vi "Begin routeguide_RouteGuide_RouteChat.vi"(8 "error in":errorcluster, 9 "contextId":T1, 11 "gRPC ID":T1) -> (0 "error out":errorcluster, 2 "Call Id Out":T1, 3 "gRPC ID out":T1)   [LabVIEW 2019, in "route_guide_client.lvlib"]
uses:
  route_guide_client.lvlib
  <vilib>/gRPC/LabVIEW gRPC Library/Shared/grpcId.ctl
  <vilib>/gRPC/LabVIEW gRPC Library/grpc-lvsupport-release.lvlib
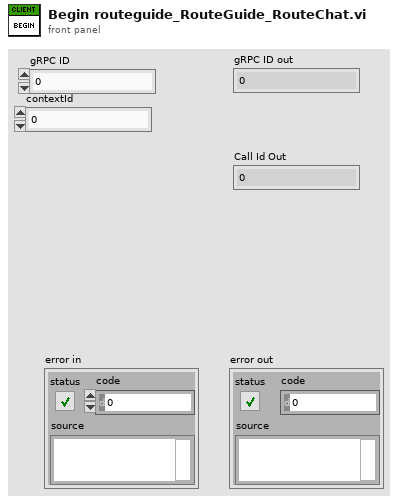
[diagram p1: front panel]
types:
  T1 = typedef "grpc-lvsupport-release.lvlib/grpcId.ctl" = u64
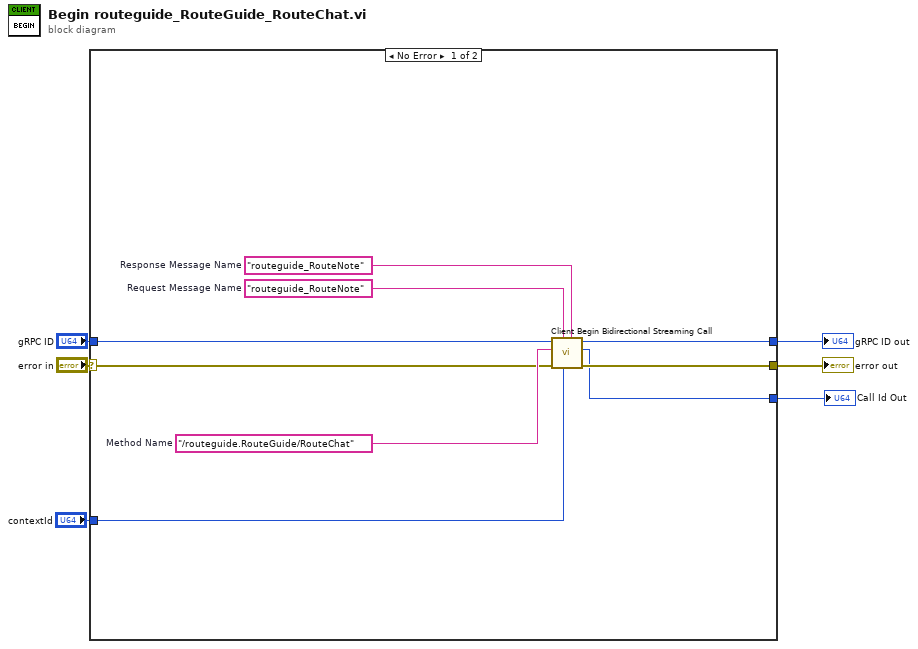
[diagram p0: block diagram]
diagram:
  n1 = case shown="No Error" "error in" {
    selector: "error in" -> [w12 w16]
    tunnel: [w11 w16] -> w5
    tunnel: "gRPC ID" -> [w10 w17]
    tunnel: [w9 w17] -> w3
    tunnel: [w8 _] -> w2
    tunnel: "contextId" -> [w7 _]
    frame No Error {
      w13 = "routeguide_RouteNote"  # Response Message Name
      w14 = "routeguide_RouteNote"  # Request Message Name
      w15 = "/routeguide.RouteGuide/RouteChat"  # Method Name
      n2 = call <vilib>:"Client Begin Bidirectional Streaming Call.vi"("Response Message Name"=w13, "contextId"=w7, "Request Message Name"=w14, "error in"=w12, "Method Name"=w15, "ClientID in"=w10) -> ("error out"=w11:errorcluster, "Call ID out"=w8:T1, "ClientID out"=w9:T1)  [unwired: 3 in]
    }
    frame Error {
    }
  }
  "error out" <- w5
  "gRPC ID out" <- w3
  "Call Id Out" <- w2
